vi "BatchModeInitialize.vi"(10 "Batch Size":dbl, 11 "client handle in":T1) -> (3 "client handle out":T1)   [LabVIEW 2020]
uses:
  <vilib>/httpClient/ClientHandle.ctl
  <vilib>/httpClient/LabVIEWHTTPClient.lvlib
  <vilib>/wsapi/NI_WebServices.lvlib
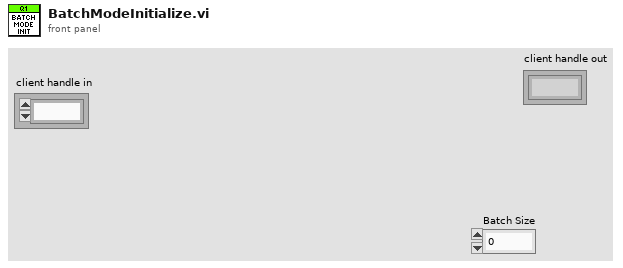
[diagram p1: front panel]
types:
  T1 = typedef "LabVIEWHTTPClient.lvlib/ClientHandle.ctl" = refnum<k1>
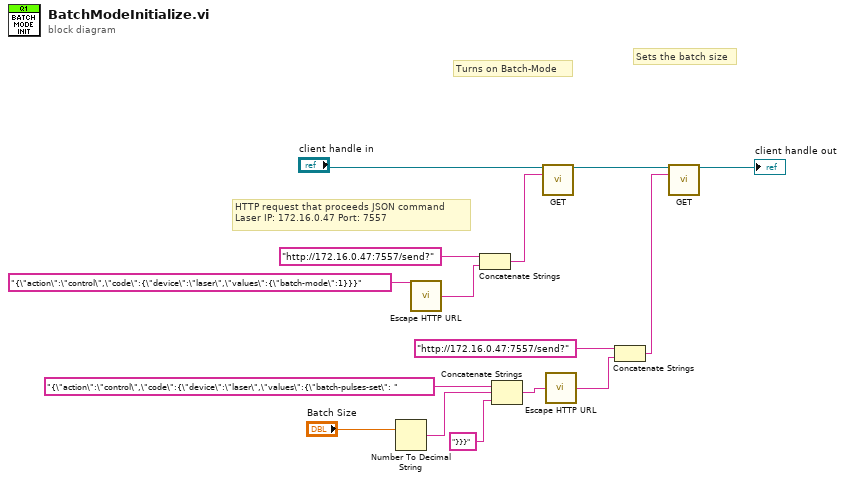
[diagram p0: block diagram]
diagram:
  # "Sets the batch size"
  # "Turns on Batch-Mode"
  # "HTTP request that proceeds JSON command\nLaser IP: 172.16.0.47 Port: 7557"
  n1 = Number To Decimal String(number="Batch Size") -> (decimal integer string=w5:string)  [unwired: 1 in]
  n2 = call <vilib>:"Escape HTTP URL.vi"("unescaped string in"="{\"action\":\"control\",\"code\":{\"device\":\"laser\",\"values\":{\"batch-mode\":1}}}" ("JSON command")) -> ("escaped string out"=w13:string)
  n3 = Concatenate Strings("http://172.16.0.47:7557/send?", w13) -> (w15:string)
  n4 = Concatenate Strings("{\"action\":\"control\",\"code\":{\"device\":\"laser\",\"values\":{\"batch-pulses-set\": " ("JSON command"), w5, "}}}" ("string")) -> (w9:string)
  n5 = call <vilib>:"GET.vi"("client handle"="client handle in", "url"=w15) -> ("client handle out"=w12:T1)  [unwired: 10 in, 3 out]
  n6 = call <vilib>:"Escape HTTP URL.vi"("unescaped string in"=w9) -> ("escaped string out"=w10:string)
  n7 = Concatenate Strings("http://172.16.0.47:7557/send?", w10) -> (w7:string)
  n8 = call <vilib>:"GET.vi"("client handle"=w12, "url"=w7) -> ("client handle out"=→"client handle out":T1)  [unwired: 10 in, 3 out]
